vi "Stop FP.vi"(8 "error in":errorcluster, 11 "Calibration UI in":refnum<class "Calibration UI.lvclass">) -> (0 "error out":errorcluster, 3 "Calibration UI out":refnum<class "Calibration UI.lvclass">)   [LabVIEW 2015, in "Calibration UI.lvclass"]
uses:
  Calibration UI.lvclass
  Calibration UI.lvclass/Calibration UI.ctl
  Reusable/GUI/GUI.lvclass
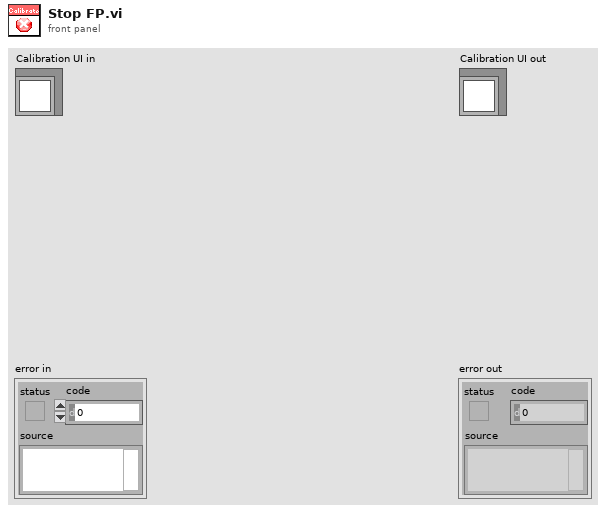
[diagram p1: front panel]
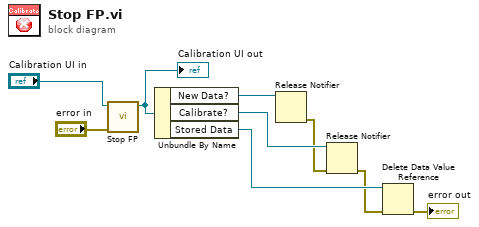
[diagram p0: block diagram]
diagram:
  n1 = call-parent "Stop FP.vi"("error in"="error in", "GUI in"="Calibration UI in") -> ("GUI out"=w1:refnum<class "Calibration UI.lvclass">)  [unwired: 8 in, 1 out]
  "Calibration UI out" <- w1
  n2 = Unbundle By Name(w1) -> ("New Data?"=w7:refnum<notifier>, "Calibrate?"=w6:refnum<notifier>, "Stored Data"=w5:refnum<data-value>)
  n3 = Release Notifier(notifier=w7) -> (error out=w4:errorcluster)  [unwired: 2 in, 2 out]
  n4 = Release Notifier(notifier=w6, error in (no error)=w4) -> (error out=w3:errorcluster)  [unwired: 1 in, 2 out]
  n5 = Delete Data Value Reference(data value reference=w5, error in=w3) -> (error out=→"error out":errorcluster)  [unwired: 1 out]
